vi "Set Amplitude Reporting Mode (Averaging) [AMP].vi"(7 "Micropulse # In":i32, 8 "error in (no error)":errorcluster, 9 "Averaging":T2 caption="Averaging (def: None)", 10 "Amplitude Mode":T1=enum."Ascan Data", 11 "Test Number":u32) -> (0 "error out":errorcluster, 5 "Micropulse # Out":i32)   [LabVIEW 2026, in "MicroPulse_Driver.lvlib"]
doc: "The specified test is set to report amplitude and TimeBase data as follows:\nMode\n=0 First peak in gate.\n=1 Largest peak in gate.\n=2 All peaks reported with TimeBase.\n=3 A-scan data reported\n(modes 2, 3 and 13 : if count n is specified the test is repeated 2n count times and averaged.)\n=10 First Threshold crossing (single Peak)\n=13 Full matrix capture.\nAscan reported from each channel in the focal law.\nFor MicroPulse 5, in this mode, the gate size is limited to 3000 sample points per channel for each transducer firing. Although gates of up to 8000 samples per channel are achievable. On LTPA the gate is limited to 8000 sample points per channel for each transducer firing.\n=30 A-scan data and all peaks reported with TimeBase reported.\n=31 All peaks reported with TimeBase for up to four hardware gates in multi-gate mode. Gates specified by GMT command.\nAveraging can be specified as a third parameter.\n=32 All peaks reported with TimeBase for up to four hardware gates in multi-gate mode. Gates specified by GMT command. Also an A-scan of the gate that encompasses the enabled peak detection gates for the test is reported.\n=33 As per mode 32 except that the A-scan data is persisted (maximum) across multiple test cycles as specified by the ACNT.\nThese A-scans can be compressed using the DCM command. No addition averaging can be specified.\nThe gates specified by the GMT command are processed on every firing. Mode 33 is intended to allow peak detection on every test whilst providing A-scans for use for display purposes with persistence. The mode is currently available in continuous inspection modes STR, STRS, STRG, STRF, FLX/FLZ and FLR. In this mode only there is a restriction of 32000 total A-scan samples across all tests in a cycle (after compression). This maximum is increased to 64000 samples if 8-bit data output is specified for A-scans via the optional second parameter of the DOF command. Mode 33 is not available in DOF 5 and 6.\nHere ‘all peaks’ means the first n peaks as defined by the PIG command.\n\nParameters:\n<Tn> : Test number. An integer value from 0 to the maximum number of tests (default maximum is 1279 tests).\nTn = 0 for all conventional tests. If the S extension is used it applies to all tests in the sweep number specified: 1-32, 0 = all sweeps.\n\n<mode> : 0 1,2,3,10,13,30,31,32 and 33\n\noptional\n[count] : Repeat count for Averaging/persistence modes\n1 to 8 for 2 to 256 averages\n\nExamples:\nAMP 1 2 3 : averages 8 firings (2^3)"
uses:
  MicroPulse_Driver.lvlib
  <instrlib>/MicroPulse/Public/Data/Datatypes/MP - averaging.ctl
  <instrlib>/MicroPulse/Public/Data/Datatypes/MP - amplitude reporting mode.ctl
  Private/MP-Registry Action-Enum.ctl
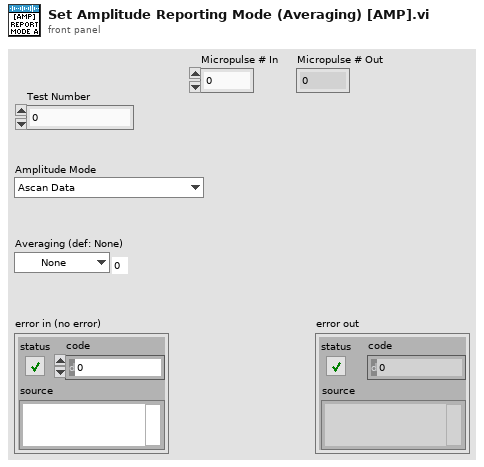
[diagram p1: front panel]
types:
  T1 = typedef "MicroPulse_Driver.lvlib/MP - amplitude reporting mode.ctl" = enum16{"1st Peak in gate", "Maximum Peak in gate", "All Peaks", "Ascan Data", "1st Threshold Crossing Peak", "Ascan + Peaks", "All Peaks for Multigate", "Peaks + Ascan for Multigate", "Peaks + P_Ascan for Multigate", "Full Matrix Capture"}
  T2 = typedef "MicroPulse_Driver.lvlib/MP - averaging.ctl" = enum16{"None", "2", "4", "8", "16", "32", "64", "128", "256"}
  T3 = typedef "MicroPulse_Driver.lvlib/MP-Registry Action-Enum.ctl" = enum16{"Read", "Add Test", "Add Command", "Add Gate Command", "Add Encoder Command", "Clear Command  List", "Set Registry", "Set System Details", "Set DOF", "Set Velocity", "Disable Asynch Reads", "Enable Asynch Reads", "Add Connection", "Disconnect", "Shutdown"}
  T4 = typedef "MicroPulse_Driver.lvlib/TCP config.ctl" = cluster{"Connection ID":refnum<k5>, "IP address":string, "host port":u16, "OC timeout":i32, "Read timeout":i32, "Write timeout":i32}
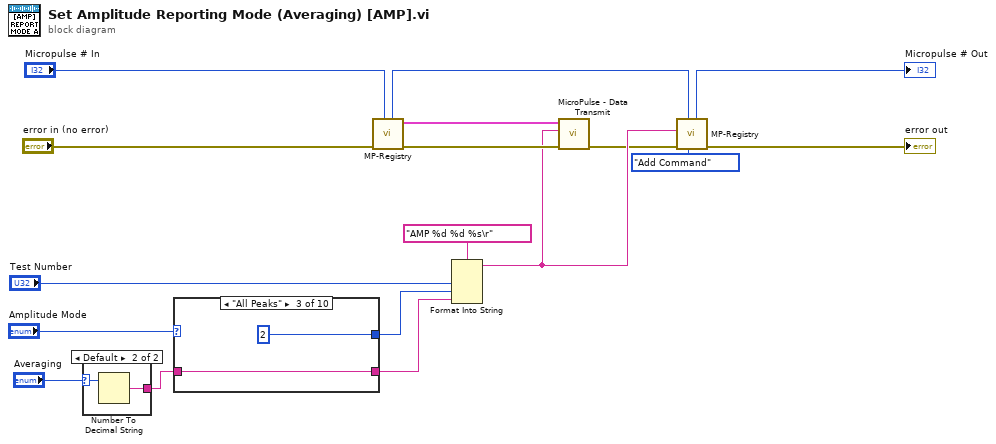
[diagram p0: block diagram]
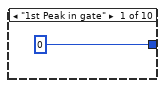
[diagram p3: hidden frame]
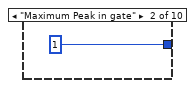
[diagram p4: hidden frame]
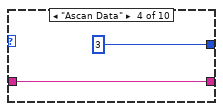
[diagram p5: hidden frame]
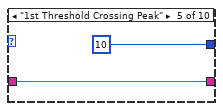
[diagram p6: hidden frame]
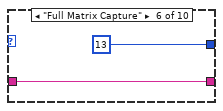
[diagram p7: hidden frame]
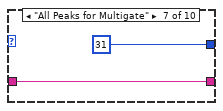
[diagram p8: hidden frame]
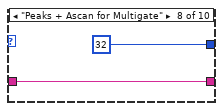
[diagram p9: hidden frame]
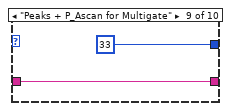
[diagram p10: hidden frame]
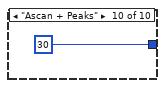
[diagram p11: hidden frame]
diagram:
  n1 = case shown="Default" "Averaging" {
    selector: "Averaging" -> [_ w18]
    tunnel: [_ w19] -> w2
    frame "None" {
    }
    frame Default {
      n2 = Number To Decimal String(number=w18) -> (decimal integer string=w19:string)  [unwired: 1 in]
    }
  }
  n3 = case shown="\"All Peaks\"" "Amplitude Mode" {
    tunnel: [0 1 2 3 10 13 31 32 33 30] -> w5
    tunnel: w2 -> [_ _ w22 w24 w26 w28 w30 w32 w34 _]
    tunnel: [_ _ w22 w24 w26 w28 w30 w32 w34 _] -> w1
    frame "1st Peak in gate" {
    }
    frame "Maximum Peak in gate" {
    }
    frame "All Peaks" {
    }
    frame "Ascan Data" {
    }
    frame "1st Threshold Crossing Peak" {
    }
    frame "Full Matrix Capture" {
    }
    frame "All Peaks for Multigate" {
    }
    frame "Peaks + Ascan for Multigate" {
    }
    frame "Peaks + P_Ascan for Multigate" {
    }
    frame "Ascan + Peaks" {
    }
  }
  n4 = call "MP-Registry.vi"("Micropulse # In"="Micropulse # In", "error in (no error)"="error in (no error)") -> ("error out"=w12:errorcluster, "TCP config"=w11:T4, "Micropulse # Out"=w7:i32)  [unwired: 6 in, 1 out]
  n5 = Format Into String(format string="AMP %d %d %s\r", "Test Number", w5, w1) -> (resulting string=w10:string)  [unwired: 2 in, 1 out]
  n6 = call "MicroPulse - Data Transmit.vi"("error in (no error)"=w12, "data"=w10, "TCP config"=w11) -> ("error out"=w8:errorcluster)  [unwired: 6 in, 2 out]
  n7 = call "MP-Registry.vi"("Action"=MP-Registry_Action-Enum."Add Command", "Micropulse # In"=w7, "error in (no error)"=w8, "Data in"=w10) -> ("error out"=→"error out":errorcluster, "Micropulse # Out"=→"Micropulse # Out":i32)  [unwired: 4 in, 2 out]
